vi "isActive.vi"(8 "error in (no error)":errorcluster, 11 "MQTT_Base in":refnum<class "MQTT_Base.lvclass">) -> (0 "error out":errorcluster, 2 "Active?":bool, 3 "MQTT_Base out":refnum<class "MQTT_Base.lvclass">)   [LabVIEW 2013, in "MQTT Base.lvlib" / "MQTT_Base.lvclass"]
uses:
  MQTT_Base.lvclass
  MQTT_Base.lvclass/MQTT_Base.ctl
  <vilib>/LabVIEW Open Source Project/MQTT Control Packets/Control Packets/ControlPacket/ControlPacket.lvclass
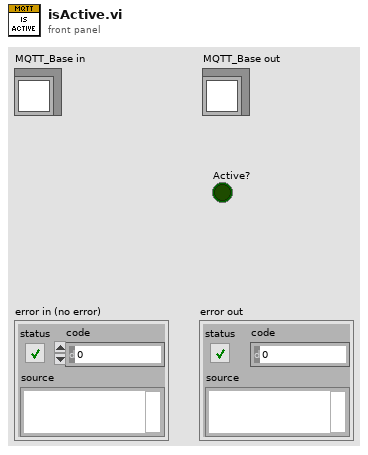
[diagram p1: front panel]
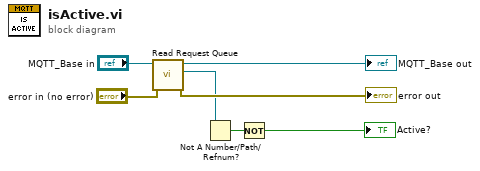
[diagram p0: block diagram]
diagram:
  n1 = call "Read Request Queue.vi"("error in (no error)"="error in (no error)", "MQTT_Base in"="MQTT_Base in") -> ("error out"=→"error out":errorcluster, "Request"=w3:refnum<queue>, "MQTT_Base out"=→"MQTT_Base out":refnum<class "MQTT_Base.lvclass">)  [unwired: 7 in]
  n2 = Not A Number/Path/Refnum?(number/path/refnum=w3) -> (NaN/Path/Refnum?=w2:bool)
  n3 = Not(x=w2) -> (.not. x?=→"Active?":bool)
